vi "WPI_CANJaguar_RecentStatus.vi"(8 "Status In":T6={"Output Percent VBus"=0.0, "Output Voltage"=0.0, "Bus Voltage"=0.0, "Current"=0.0, "Temperature"=0.0, "Position"=0.0, "Speed"=0.0, "Limits"={"Forward Limit"=TRUE, "Reverse Limit"=TRUE, "Forward Soft Limit"=TRUE, "Reverse Soft Limit"=TRUE, "Sticky Forward Limit"=TRUE, "Sticky Reverse Limit"=TRUE, "Sticky Forward Soft Limit"=TRUE, "Sticky Reverse Soft Limit"=TRUE}, "Faults"={"Current Fault"=FALSE, "Temperature Fault"=FALSE, "Bus Voltage Fault"=FALSE, "Gate Driver Fault"=FALSE, "Comm Fault"=FALSE}, "Fault Counters"={"Current Faults"=0, "Temperature Faults"=0, "Bus Voltage Faults"=0, "Gate Driver Faults"=0, "Comm Faults"=0, "CAN Status"=0, "CAN RX Errors"=0, "CAN TX Errors"=0}, "Power Cycle"=FALSE} {"Fault Counters"."CAN Status" format="%.0x"}, 9 "Update":bool, 10 "Fields":T5[](array[typedef]), 11 "CAN Jaguar Ref":T1={"DeviceStatus"={"status"=FALSE, "code"=0, "source"=""}, "Type"=enum."PWM", "PWM"={"PWM Channel"=enum."PWM 1", "DeadBand"={"Name"="", "maxPositivePwm"=0, "minPositivePwm"=0, "centerPwm"=0, "maxNegativePwm"=0, "minNegativePwm"=0, "angularRange"=0}}, "CAN"={"Device Number"=0, "SetOutput VI Ref"=variant(enum8{"Percent VBus", "Current", "Speed", "Position", "Voltage"} enum."Percent VBus"), "GetOutput VI Ref"=variant(refnum<k1> refnum), "Enable VI Ref"=variant(dbl 12.0), "Disable VI Ref"=variant(enum8{"Percent VBus", "Speed", "Position", "Slave", "Unchanged / Invalid", "Voltage Compensation", "Current", "Motion Profile"} enum."Percent VBus"), "Data"=variant}, "Invert"=FALSE}) -> (0 "Status Out":T6={"Output Percent VBus"=0.0, "Output Voltage"=0.0, "Bus Voltage"=0.0, "Current"=0.0, "Temperature"=0.0, "Position"=0.0, "Speed"=0.0, "Limits"={"Forward Limit"=TRUE, "Reverse Limit"=TRUE, "Forward Soft Limit"=TRUE, "Reverse Soft Limit"=TRUE, "Sticky Forward Limit"=TRUE, "Sticky Reverse Limit"=TRUE, "Sticky Forward Soft Limit"=TRUE, "Sticky Reverse Soft Limit"=TRUE}, "Faults"={"Current Fault"=FALSE, "Temperature Fault"=FALSE, "Bus Voltage Fault"=FALSE, "Gate Driver Fault"=FALSE, "Comm Fault"=FALSE}, "Fault Counters"={"Current Faults"=0, "Temperature Faults"=0, "Bus Voltage Faults"=0, "Gate Driver Faults"=0, "Comm Faults"=0, "CAN Status"=0, "CAN RX Errors"=0, "CAN TX Errors"=0}, "Power Cycle"=FALSE} {"Fault Counters"."CAN Status" format="%.0x"})   [LabVIEW 2016]
uses:
  <vilib>/Rock Robotics/WPI/ThirdParty/CanMotor/CAN Jaguar/SubVIs/WPI_CANJaguar_Status.ctl
  <vilib>/Rock Robotics/WPI/ThirdParty/CanMotor/CAN Jaguar/SubVIs/WPI_CAN_PeriodicStatusIDs.ctl
  <vilib>/Rock Robotics/WPI/MotorControl/WPI_MotorControlDeviceRef.ctl
  <vilib>/Rock Robotics/WPI/MotorControl/WPI_MotorControlType.ctl
  <vilib>/Rock Robotics/SystemInterfaces/DIO/FPGA_DIOPWMChannel.ctl
  <vilib>/Rock Robotics/WPI/PWM/WPI_PWMDeadband.ctl
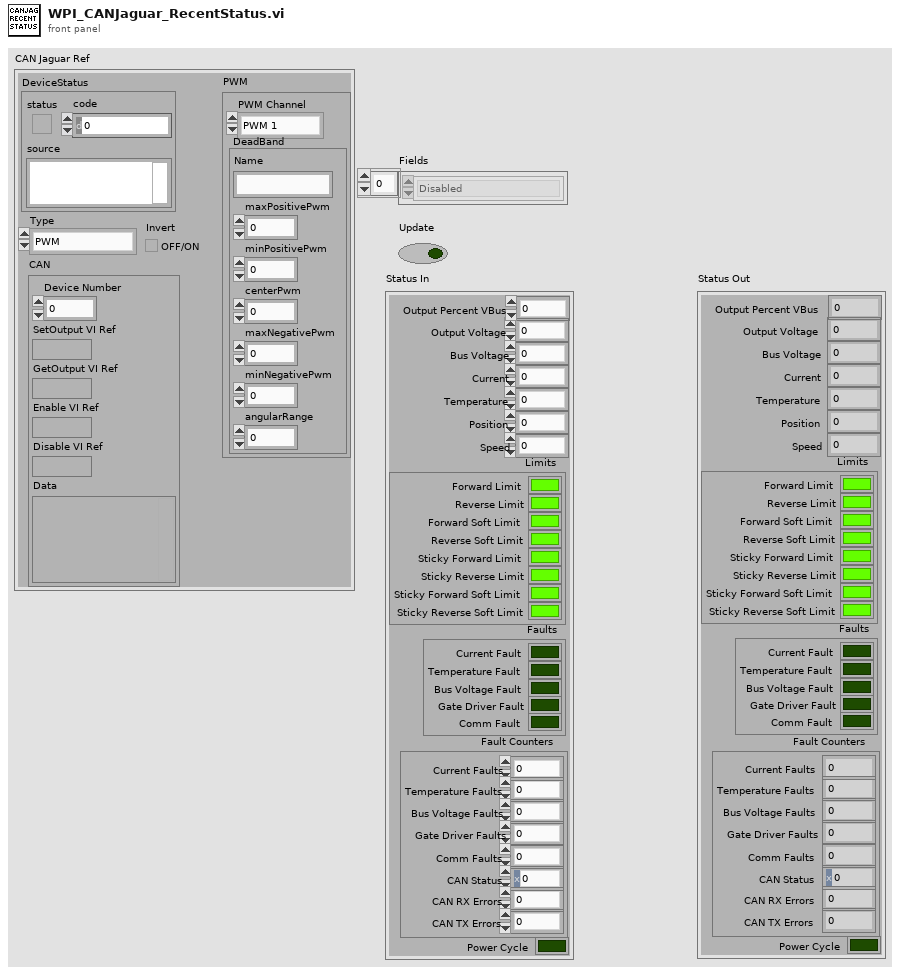
[diagram p1: front panel]
types:
  T1 = typedef "WPI_MotorControlDeviceRef.ctl" = cluster{"DeviceStatus":errorcluster, "Type":T2, "PWM":cluster{"PWM Channel":T3, "DeadBand":T4}, "CAN":cluster{"Device Number":u8, "SetOutput VI Ref":variant, "GetOutput VI Ref":variant, "Enable VI Ref":variant, "Disable VI Ref":variant, "Data":variant}, "Invert":bool}
  T2 = typedef "WPI_MotorControlType.ctl" = enum16{"PWM", "CAN"}
  T3 = typedef "FPGA_DIOPWMChannel.ctl" = enum8{"PWM 0", "PWM 1", "PWM 2", "PWM 3", "PWM 4", "PWM 5", "PWM 6", "PWM 7", "PWM 8", "PWM 9", "PWM MXP 0", "PWM MXP 1", "PWM MXP 2", "PWM MXP 3", "PWM MXP 4", "PWM MXP 5", "PWM MXP 6", "PWM MXP 7", "PWM MXP 8", "PWM MXP 9", "Invalid"}
  T4 = typedef "WPI_PWMDeadband.ctl" = cluster{"Name":string, "maxPositivePwm":i32, "minPositivePwm":i32, "centerPwm":i32, "maxNegativePwm":i32, "minNegativePwm":i32, "angularRange":u16}
  T5 = typedef "WPI_CAN_PeriodicStatusIDs.ctl" = enum16{"Disabled", "Percent VBus Out (Byte 0)", "Percent VBus Out (Byte 1)", "VBus (Byte 0)", "VBus (Byte 1)", "Current (Byte 0)", "Current (Byte 1)", "Temperature (Byte 0)", "Temperature (Byte 1)", "Position (Byte 0)", "Position (Byte 1)", "Position (Byte 2)", "Position (Byte 3)", "Speed (Byte 0)", "Speed (Byte 1)", "Speed (Byte 2)", "Speed (Byte 3)", "Limit Switches (No Clear)", "Limit Switches (Clear)", "Faults", "Sticky Faults (No Clear)", "Sticky Faults (Clear)", "Volts Out (Byte 0)", "Volts Out (Byte 1)", "Current Fault Counter", "Temperature Fault Counter", "VBus Fault Counter", "Gate Driver Fault Counter", "Comm Fault Counter", "CANSTS", "CANERR (Byte 0)", "CANERR (Byte 1)", "Power Cycle"}
  T6 = typedef "WPI_CANJaguar_Status.ctl" = cluster{"Output Percent VBus":dbl, "Output Voltage":dbl, "Bus Voltage":dbl, "Current":dbl, "Temperature":dbl, "Position":dbl, "Speed":dbl, "Limits":cluster{"Forward Limit":bool, "Reverse Limit":bool, "Forward Soft Limit":bool, "Reverse Soft Limit":bool, "Sticky Forward Limit":bool, "Sticky Reverse Limit":bool, "Sticky Forward Soft Limit":bool, "Sticky Reverse Soft Limit":bool}, "Faults":cluster{"Current Fault":bool, "Temperature Fault":bool, "Bus Voltage Fault":bool, "Gate Driver Fault":bool, "Comm Fault":bool}, "Fault Counters":cluster{"Current Faults":u8, "Temperature Faults":u8, "Bus Voltage Faults":u8, "Gate Driver Faults":u8, "Comm Faults":u8, "CAN Status":u8, "CAN RX Errors":u8, "CAN TX Errors":u8}, "Power Cycle":bool}
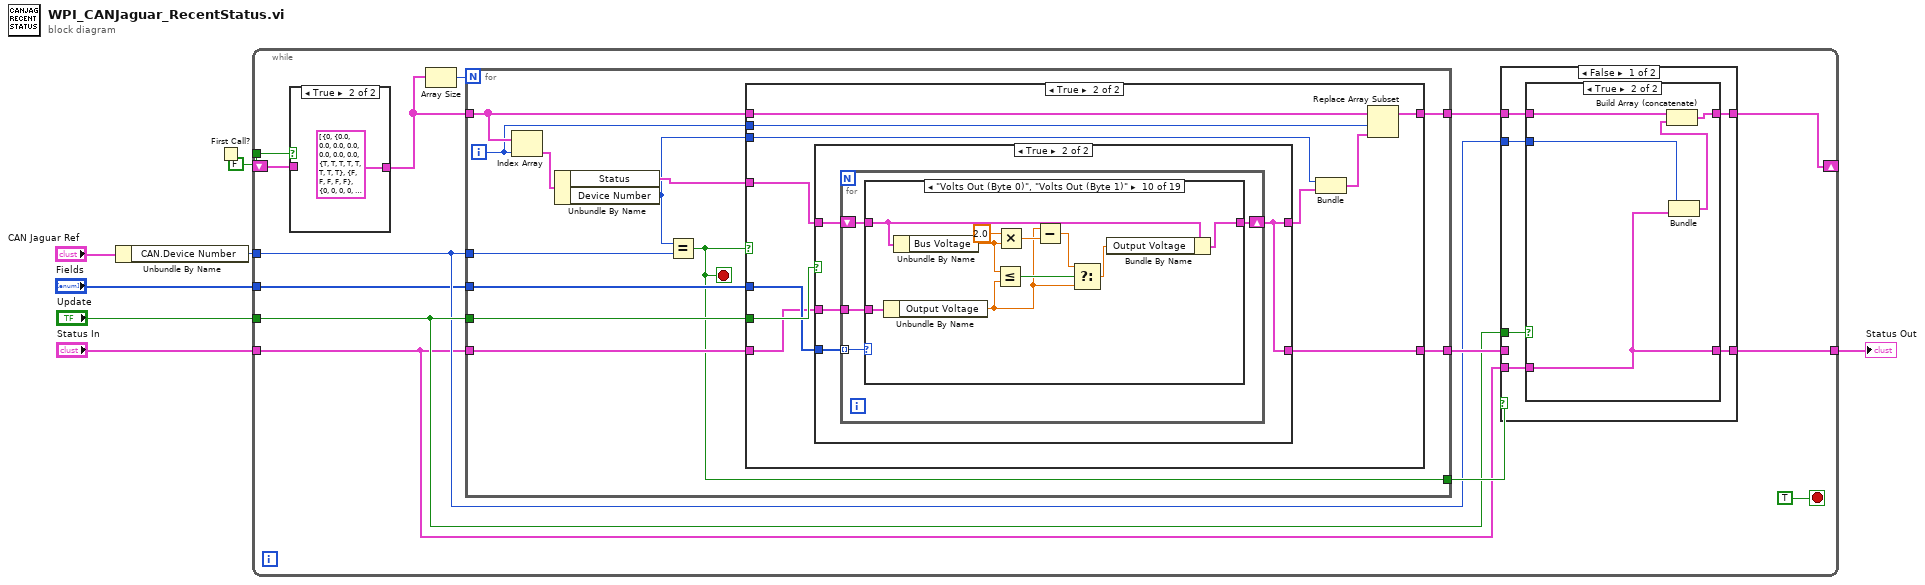
[diagram p0: block diagram]
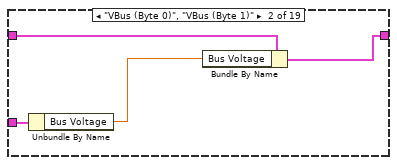
[diagram p7: hidden frame]
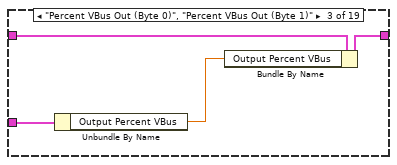
[diagram p8: hidden frame]
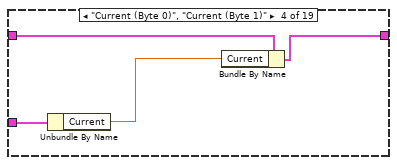
[diagram p9: hidden frame]
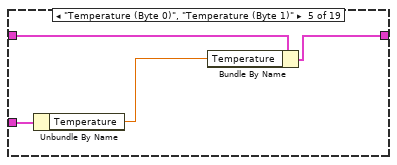
[diagram p10: hidden frame]
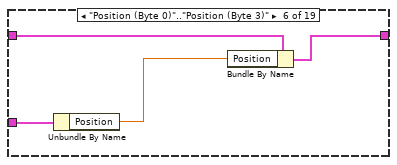
[diagram p11: hidden frame]
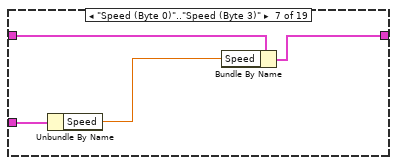
[diagram p12: hidden frame]
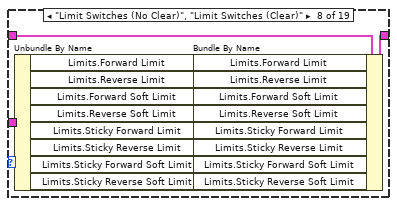
[diagram p13: hidden frame]
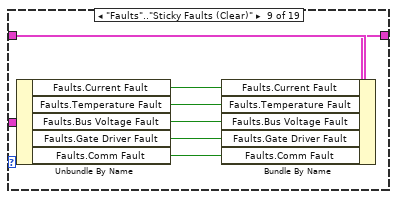
[diagram p14: hidden frame]
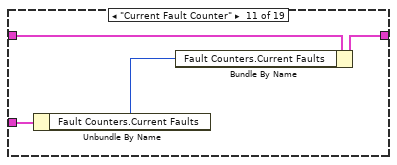
[diagram p15: hidden frame]
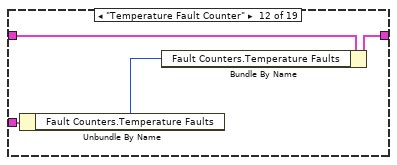
[diagram p16: hidden frame]
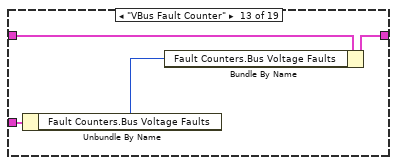
[diagram p17: hidden frame]
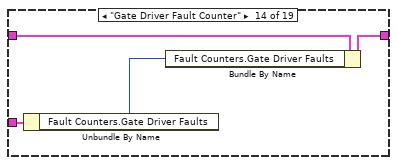
[diagram p18: hidden frame]
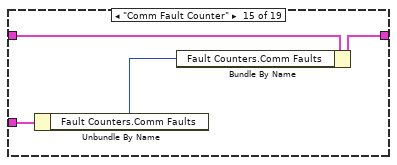
[diagram p19: hidden frame]
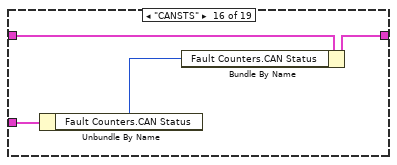
[diagram p20: hidden frame]
diagram:
  n1 = Unbundle By Name("CAN Jaguar Ref") -> ("CAN.Device Number"=w3:u8)
  n2 = First Call?() -> ()  [unwired: 1 out]
  n3 = while {
    tunnel: "Status In" -> [w9]
    tunnel: "Update" -> [w11]
    tunnel: "Fields" -> [w8]
    tunnel: FALSE ("First Call?: T/F") -> [w20]
    tunnel: [w15] -> w2
    shift-right: [w13] -> _
    shift-left: _ -> [w19]
    tunnel: w3 -> [w10]
    stop <- TRUE stop-if-true
    n4 = case shown="True" w20 {
      tunnel: w19 -> [w159 _]
      tunnel: [w159 cluster{"Device Number":u8, "Status":T6}[] [{"Device Number"=0, "Status"={"Output Percent VBus"=0.0, "Output Voltage"=0.0, "Bus Voltage"=0.0, "Current"=0.0, "Temperature"=0.0, "Position"=0.0, "Speed"=0.0, "Limits"={"Forward Limit"=TRUE, "Reverse Limit"=TRUE, "Forward Soft Limit"=TRUE, "Reverse Soft Limit"=TRUE, "Sticky Forward Limit"=TRUE, "Sticky Reverse Limit"=TRUE, "Sticky Forward Soft Limit"=TRUE, "Sticky Reverse Soft Limit"=TRUE}, "Faults"={"Current Fault"=FALSE, "Temperature Fault"=FALSE, "Bus Voltage Fault"=FALSE, "Gate Driver Fault"=FALSE, "Comm Fault"=FALSE}, "Fault Counters"={"Current Faults"=0, "Temperature Faults"=0, "Bus Voltage Faults"=0, "Gate Driver Faults"=0, "Comm Faults"=0, "CAN Status"=0, "CAN RX Errors"=0, "CAN TX Errors"=0}, "Power Cycle"=FALSE}}]] -> w17
      frame False {
      }
      frame True {
      }
    }
    n5 = Array Size(array=w17) -> (size(s)=w18:i32)
    n6 = for {
      N: w18 -> [_]
      tunnel: w11 -> [w47]
      tunnel: w8 -> [w46]
      tunnel: [w40] -> w12
      tunnel: w17 -> [w39]
      tunnel: w10 -> [w41]
      tunnel: [w38] -> w16
      tunnel: w9 -> [w45]
      tunnel: [w44] -> w14
      i -> [w37]
      stop <- w38 stop-if-true
      n7 = Index Array(array=w39, index=w37) -> (element=w43:cluster{"Device Number":u8, "Status":T6})
      n8 = Unbundle By Name(w43) -> ("Status"=w42:T6, "Device Number"=w36:u8)
      n9 = Equal?(x=w36, y=w41) -> (x = y?=w38:bool)
      n10 = case shown="True" w38 {
        tunnel: w47 -> [_ w54]
        tunnel: w46 -> [_ w51]
        tunnel: w45 -> [_ w50]
        tunnel: [_ w49] -> w44
        tunnel: w42 -> [_ w53]
        tunnel: [w48 w58] -> w40
        tunnel: w39 -> [w48 w59]
        tunnel: w37 -> [_ w57]
        tunnel: w36 -> [_ w56]
        frame False {
        }
        frame True {
          n11 = case shown="True" w54 {
            tunnel: w50 -> [_ w61]
            tunnel: [w60 w62] -> w49
            tunnel: w53 -> [w60 w63]
            tunnel: [w60 w62] -> w52
            tunnel: w51 -> [_ w64]
            frame False {
            }
            frame True {
              n12 = for {
                tunnel: w64 -> [w68] mode=indexing
                shift-right: [w65] -> w62
                shift-left: w63 -> [w66]
                tunnel: w61 -> [w67]
                n13 = case shown="\"Volts Out (Byte 0)\", \"Volts Out (Byte 1)\"" w68 {
                  tunnel: w67 -> [_ w71 w75 w80 w84 w88 w92 w103 w111 w122 w125 w129 w133 w137 w141 w145 w149 w153 w157]
                  tunnel: w66 -> [w69 w73 w77 w79 w83 w87 w91 w102 w110 w120 w123 w127 w131 w135 w139 w143 w147 w151 w155]
                  tunnel: [w69 w72 w76 w78 w82 w86 w90 w101 w109 w121 w124 w128 w132 w136 w140 w144 w148 w152 w156] -> w65
                  frame "Disabled", Default {
                  }
                  frame "VBus (Byte 0)", "VBus (Byte 1)" {
                    n14 = Unbundle By Name(w71) -> ("Bus Voltage"=w70:dbl)
                    n15 = Bundle By Name(cluster=w73, "Bus Voltage"=w70) -> (w72:T6)
                  }
                  frame "Percent VBus Out (Byte 0)", "Percent VBus Out (Byte 1)" {
                    n16 = Unbundle By Name(w75) -> ("Output Percent VBus"=w74:dbl)
                    n17 = Bundle By Name(cluster=w77, "Output Percent VBus"=w74) -> (w76:T6)
                  }
                  frame "Current (Byte 0)", "Current (Byte 1)" {
                    n18 = Unbundle By Name(w80) -> ("Current"=w81:dbl)
                    n19 = Bundle By Name(cluster=w79, "Current"=w81) -> (w78:T6)
                  }
                  frame "Temperature (Byte 0)", "Temperature (Byte 1)" {
                    n20 = Unbundle By Name(w84) -> ("Temperature"=w85:dbl)
                    n21 = Bundle By Name(cluster=w83, "Temperature"=w85) -> (w82:T6)
                  }
                  frame "Position (Byte 0)".."Position (Byte 3)" {
                    n22 = Unbundle By Name(w88) -> ("Position"=w89:dbl)
                    n23 = Bundle By Name(cluster=w87, "Position"=w89) -> (w86:T6)
                  }
                  frame "Speed (Byte 0)".."Speed (Byte 3)" {
                    n24 = Unbundle By Name(w92) -> ("Speed"=w93:dbl)
                    n25 = Bundle By Name(cluster=w91, "Speed"=w93) -> (w90:T6)
                  }
                  frame "Limit Switches (No Clear)", "Limit Switches (Clear)" {
                    n26 = Unbundle By Name(w103) -> ("Limits.Forward Limit"=w104:bool, "Limits.Reverse Limit"=w100:bool, "Limits.Forward Soft Limit"=w99:bool, "Limits.Reverse Soft Limit"=w98:bool, "Limits.Sticky Forward Limit"=w97:bool, "Limits.Sticky Reverse Limit"=w96:bool, "Limits.Sticky Forward Soft Limit"=w95:bool, "Limits.Sticky Reverse Soft Limit"=w94:bool)
                    n27 = Bundle By Name(cluster=w102, "Limits.Forward Limit"=w104, "Limits.Reverse Limit"=w100, "Limits.Forward Soft Limit"=w99, "Limits.Reverse Soft Limit"=w98, "Limits.Sticky Forward Limit"=w97, "Limits.Sticky Reverse Limit"=w96, "Limits.Sticky Forward Soft Limit"=w95, "Limits.Sticky Reverse Soft Limit"=w94) -> (w101:T6)
                  }
                  frame "Faults".."Sticky Faults (Clear)" {
                    n28 = Unbundle By Name(w111) -> ("Faults.Current Fault"=w112:bool, "Faults.Temperature Fault"=w108:bool, "Faults.Bus Voltage Fault"=w107:bool, "Faults.Gate Driver Fault"=w106:bool, "Faults.Comm Fault"=w105:bool)
                    n29 = Bundle By Name(cluster=w110, "Faults.Current Fault"=w112, "Faults.Temperature Fault"=w108, "Faults.Bus Voltage Fault"=w107, "Faults.Gate Driver Fault"=w106, "Faults.Comm Fault"=w105) -> (w109:T6)
                  }
                  frame "Volts Out (Byte 0)", "Volts Out (Byte 1)" {
                    n30 = Unbundle By Name(w122) -> ("Output Voltage"=w114:dbl)
                    n31 = Unbundle By Name(w120) -> ("Bus Voltage"=w117:dbl)
                    n32 = Less Or Equal?(x=w117, y=w114) -> (x <= y?=w119:bool)
                    n33 = Multiply(x=2.0, y=w117) -> (x*y=w115:dbl)
                    n34 = Subtract(x=w114, y=w115) -> (x-y=w113:dbl)
                    n35 = Select(t=w113, s=w119, f=w114) -> (s? t:f=w118:dbl)
                    n36 = Bundle By Name(cluster=w120, "Output Voltage"=w118) -> (w121:T6)
                  }
                  frame "Current Fault Counter" {
                    n37 = Unbundle By Name(w125) -> ("Fault Counters.Current Faults"=w126:u8)
                    n38 = Bundle By Name(cluster=w123, "Fault Counters.Current Faults"=w126) -> (w124:T6)
                  }
                  frame "Temperature Fault Counter" {
                    n39 = Unbundle By Name(w129) -> ("Fault Counters.Temperature Faults"=w130:u8)
                    n40 = Bundle By Name(cluster=w127, "Fault Counters.Temperature Faults"=w130) -> (w128:T6)
                  }
                  frame "VBus Fault Counter" {
                    n41 = Unbundle By Name(w133) -> ("Fault Counters.Bus Voltage Faults"=w134:u8)
                    n42 = Bundle By Name(cluster=w131, "Fault Counters.Bus Voltage Faults"=w134) -> (w132:T6)
                  }
                  frame "Gate Driver Fault Counter" {
                    n43 = Unbundle By Name(w137) -> ("Fault Counters.Gate Driver Faults"=w138:u8)
                    n44 = Bundle By Name(cluster=w135, "Fault Counters.Gate Driver Faults"=w138) -> (w136:T6)
                  }
                  frame "Comm Fault Counter" {
                    n45 = Unbundle By Name(w141) -> ("Fault Counters.Comm Faults"=w142:u8)
                    n46 = Bundle By Name(cluster=w139, "Fault Counters.Comm Faults"=w142) -> (w140:T6)
                  }
                  frame "CANSTS" {
                    n47 = Unbundle By Name(w145) -> ("Fault Counters.CAN Status"=w146:u8)
                    n48 = Bundle By Name(cluster=w143, "Fault Counters.CAN Status"=w146) -> (w144:T6)
                  }
                  frame "CANERR (Byte 0)" {
                    n49 = Unbundle By Name(w149) -> ("Fault Counters.CAN RX Errors"=w150:u8)
                    n50 = Bundle By Name(cluster=w147, "Fault Counters.CAN RX Errors"=w150) -> (w148:T6)
                  }
                  frame "CANERR (Byte 1)" {
                    n51 = Unbundle By Name(w153) -> ("Fault Counters.CAN TX Errors"=w154:u8)
                    n52 = Bundle By Name(cluster=w151, "Fault Counters.CAN TX Errors"=w154) -> (w152:T6)
                  }
                  frame "Power Cycle" {
                    n53 = Unbundle By Name(w157) -> ("Power Cycle"=w158:bool)
                    n54 = Bundle By Name(cluster=w155, "Power Cycle"=w158) -> (w156:T6)
                  }
                }
              }
            }
          }
          n55 = Bundle("Device Number"=w56, "Status"=w52) -> (w55:cluster{"Device Number":u8, "Status":T6})  [unwired: 1 in]
          n56 = Replace Array Subset(array=w59, new element=w55, index=w57) -> (w58:cluster{"Device Number":u8, "Status":T6}[])
        }
      }
    }
    n57 = case shown="False" w16 {
      tunnel: [w23 w35] -> w15
      tunnel: w14 -> [_ w35]
      tunnel: [w25 w34] -> w13
      tunnel: w12 -> [w26 w34]
      tunnel: w11 -> [w27 _]
      tunnel: w10 -> [w22 _]
      tunnel: w9 -> [w24 _]
      frame False {
        n58 = case shown="True" w27 {
          tunnel: w26 -> [w28 w33]
          tunnel: [w28 w32] -> w25
          tunnel: w24 -> [_ w29]
          tunnel: [_ w29] -> w23
          tunnel: w22 -> [_ w31]
          frame False {
          }
          frame True {
            n59 = Bundle("Device Number"=w31, "Status In"=w29) -> (w30:cluster{"Device Number":u8, "Status In":T6})  [unwired: 1 in]
            n60 = Build Array (concatenate)(w33, w30) -> (w32:cluster{"Device Number":u8, "Status In":T6}[])
          }
        }
      }
      frame True {
      }
    }
  }
  "Status Out" <- w2
